vi "XW_Tutu_Chevray.vi"() -> (5 "Plug in titles":string[](array[string]), 7 "Plug in values":string[](array[string]))   [LabVIEW 2010]
uses:
  Globals/Meas_global.vi
  Controls/Analysis_type_Enum.ctl
  Controls/In_Range.ctl
  <vilib>/Utility/file.llb/Read From Spreadsheet File (string).vi
panel:
  out "Third":dbl format="%#.3f"
  out "Filename":string
  out "Third Component":path
  out "Info index":i32
  out "Log Row":i32
  out "2nd Comp":string
  out "1st Comp":string
  out "Iterations":i32
  out "Results table":string[][](table)
  out "Psi 2":dbl=-999.0 format="%.2f"
  out "Psi 1":dbl=-999.0 format="%.2f"
  out "UW":bool
  out "Indicies":i32[](array[numeric])
  in  "constants":T1={"u'/U"=0.5, "v'/U"=0.4, "w'/U"=0.4, "rho"=0.5, "alpha1"=0.0, "alpha2"=0.0} {"alpha2" format="%.2f"; "alpha1" format="%.2f"; "rho" format="%.2f"; "w'/U" format="%.2f"; "v'/U" format="%.2f"; "u'/U" format="%.2f"}
  in  "u*, v* limits":T2={"u* low"=0.4, "u* high"=1.8, "v* low"=-0.6, "v* high"=0.8} {"v* high" format="%.2f"; "v* low" format="%.2f"; "u* high" format="%.2f"; "u* low" format="%.2f"}
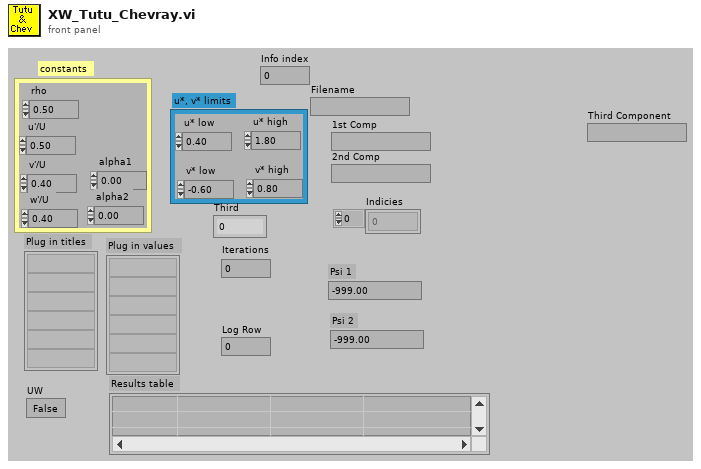
[diagram p1: front panel]
types:
  T1 = cluster{"u'/U":dbl, "v'/U":dbl, "w'/U":dbl, "rho":dbl, "alpha1":dbl, "alpha2":dbl}
  T2 = cluster{"u* low":dbl, "u* high":dbl, "v* low":dbl, "v* high":dbl}
  T3 = typedef "Correlation_cluster.ctl" = cluster{"U inst":string, "W inst":string, "uw":dbl, "uw/u'w'":dbl, "u^2w":dbl, "uw^2":dbl, "uw^3":dbl, "u^3w":dbl, "u^2w^2":dbl}
  T4 = typedef "Velocity_cluster.ctl" = cluster{"Name":string, "U":dbl, "u^2":dbl, "u^3/(u^2)^(1.5)":dbl, "u^4/(u^2)^2 -3":dbl, "% u'/U":dbl, "Mean % Err":dbl, "u^4":dbl}
  T5 = typedef "Analysis_type_cluster.ctl" = cluster{"Analysis type":T6, "Indicies":i32[], "Name":string, "Inst Array":T7, "Info index":i32}
  T6 = typedef "Analysis_type_Enum.ctl" = enum16{"Slow Response", "Fast Response", "Weighted Fast Response", "Fast FID", "Weighted Fast FID", "Cross Wire", "Weighted Cross Wire", "Weighted LDA"}
  T7 = typedef "Instrument_Array.ctl" = enum16{"PWA", "LDA", "Analogue"}
  T8 = typedef "In_Range.ctl" = enum16{"%", "±", "% & ±"}
  T9 = enum16{"Save no data", "Save data in new files", "Save data in existing files"}
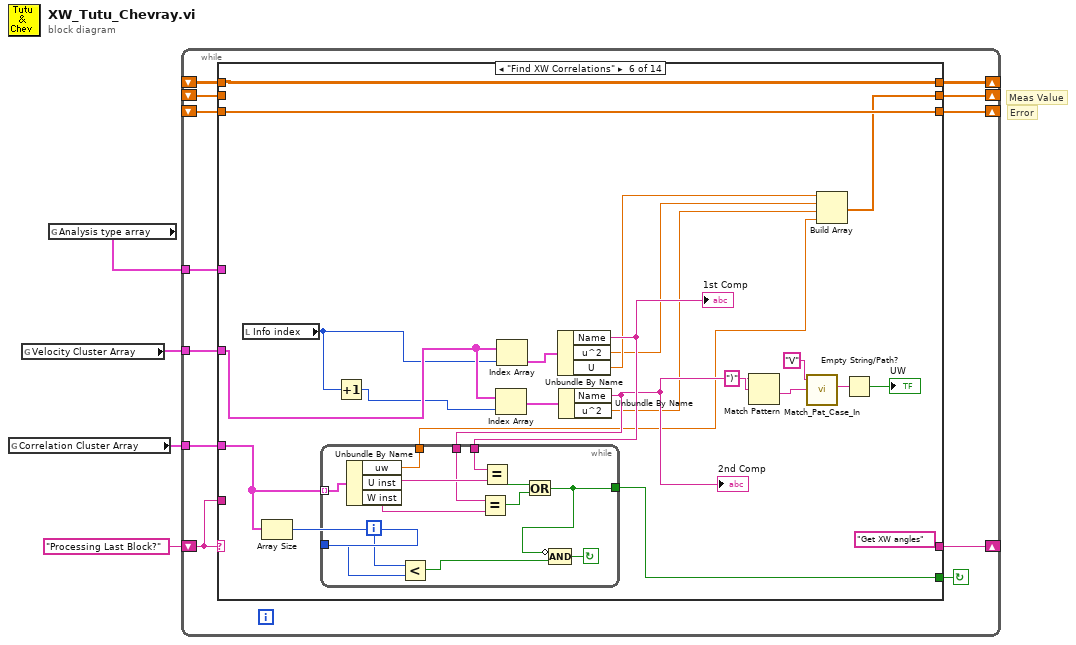
[diagram p0: block diagram]
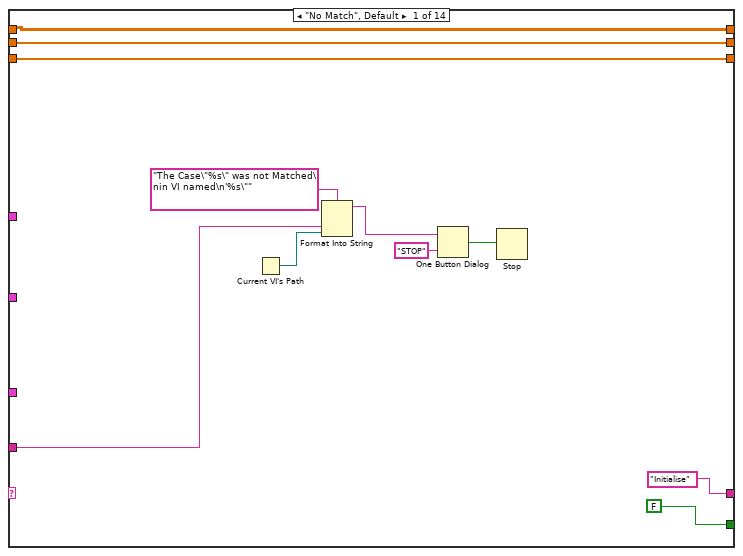
[diagram p2: hidden frame]
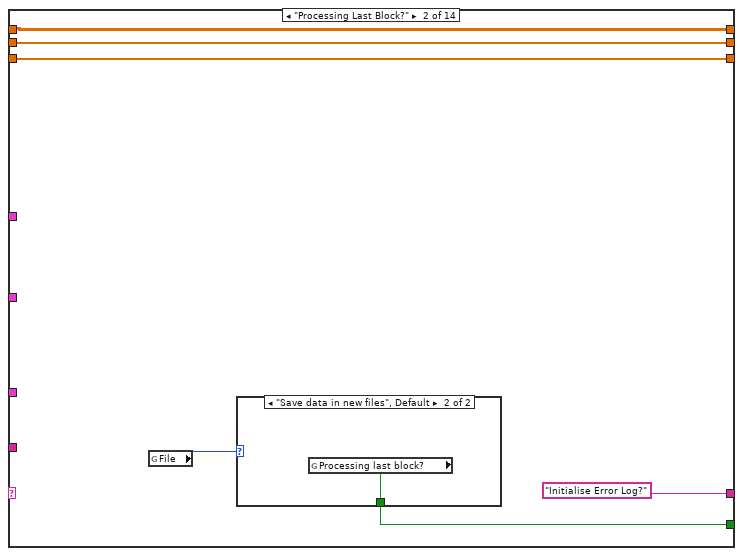
[diagram p3: hidden frame]
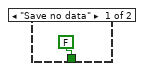
[diagram p4: hidden frame]
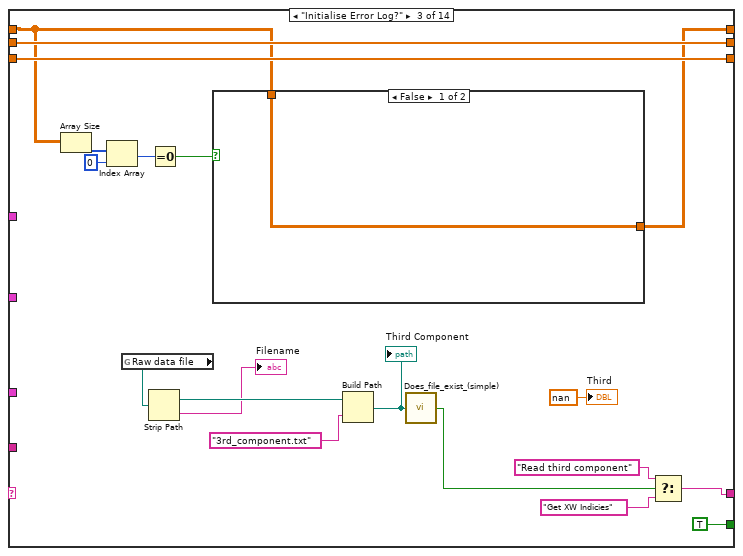
[diagram p5: hidden frame]
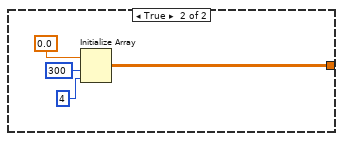
[diagram p6: hidden frame]
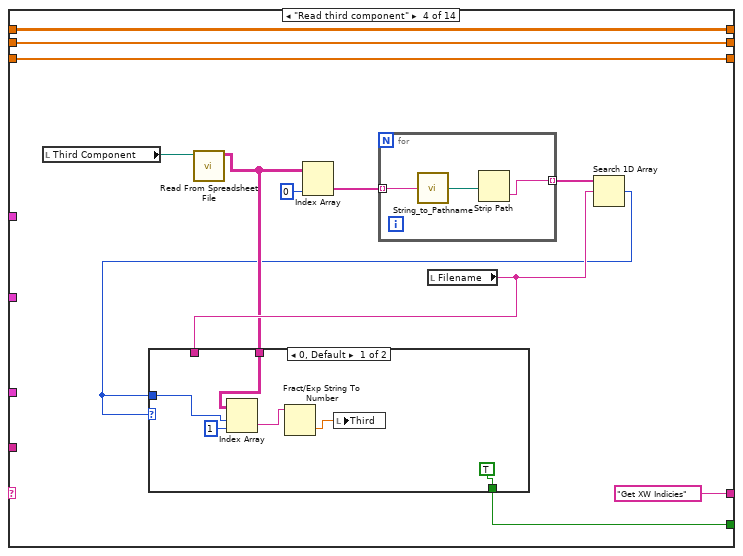
[diagram p7: hidden frame]
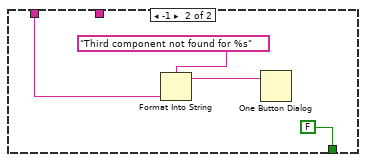
[diagram p8: hidden frame]
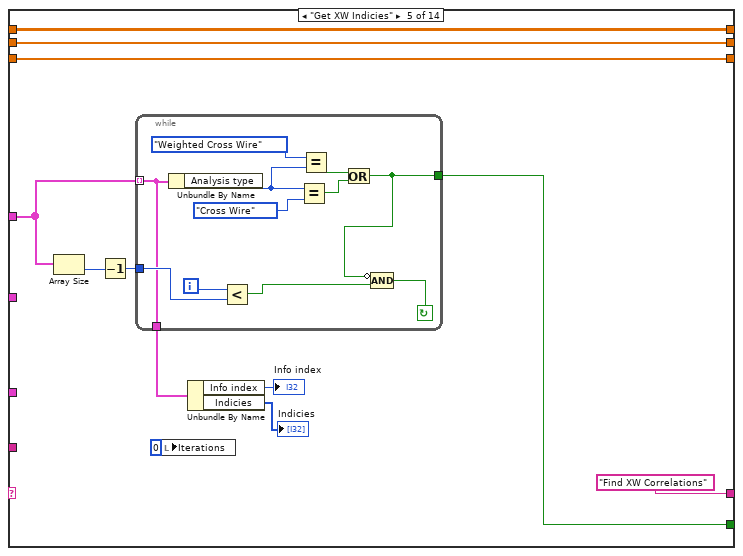
[diagram p9: hidden frame]
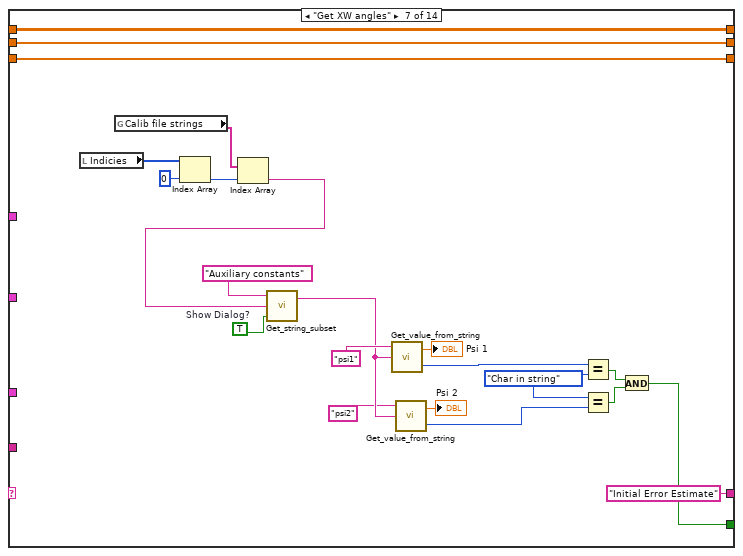
[diagram p10: hidden frame]
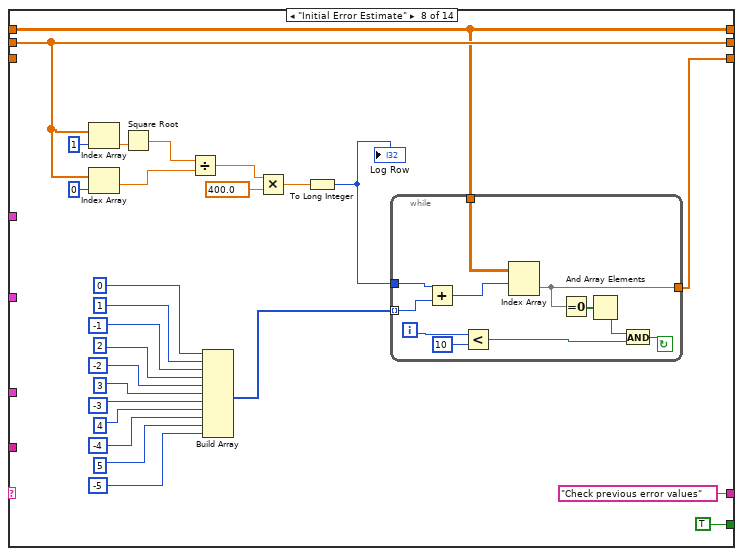
[diagram p11: hidden frame]
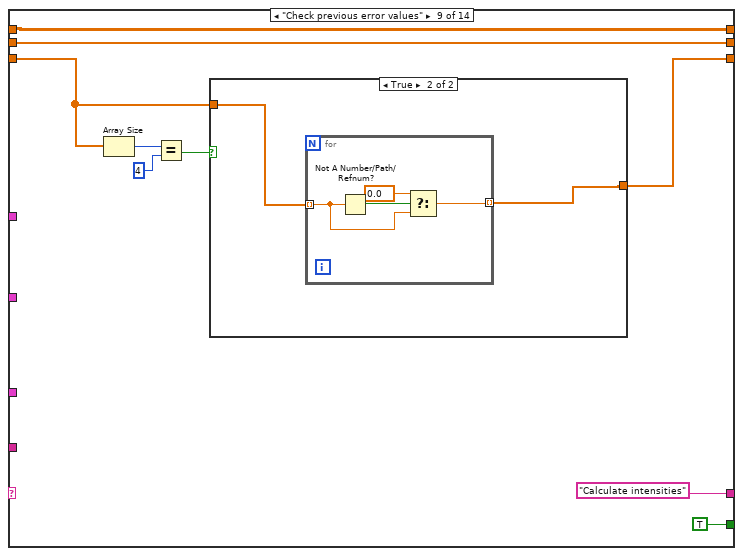
[diagram p12: hidden frame]
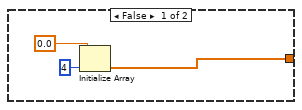
[diagram p13: hidden frame]
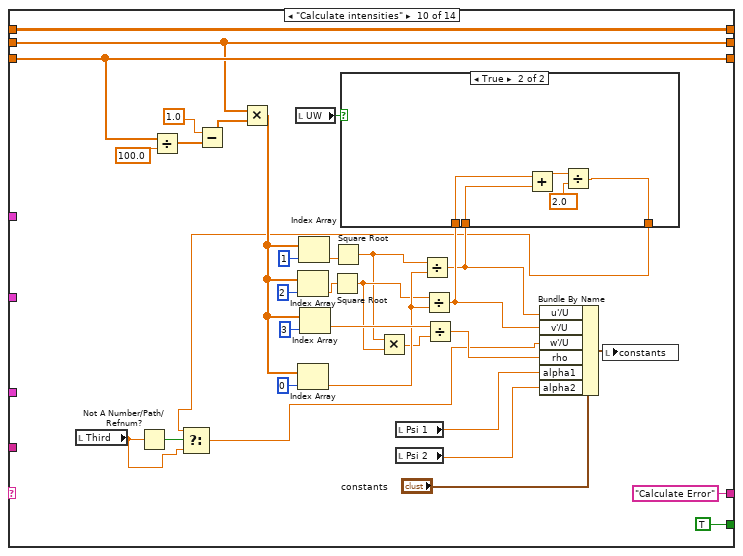
[diagram p14: hidden frame]
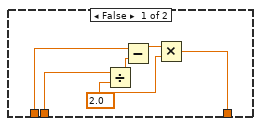
[diagram p15: hidden frame]
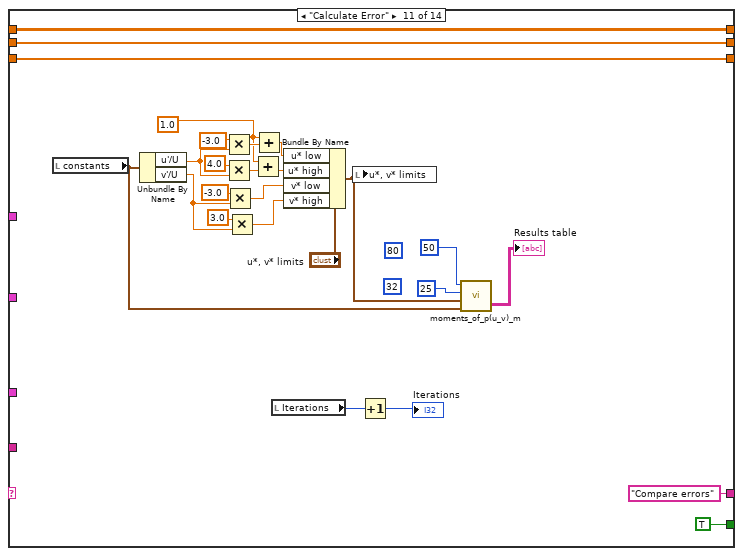
[diagram p16: hidden frame]
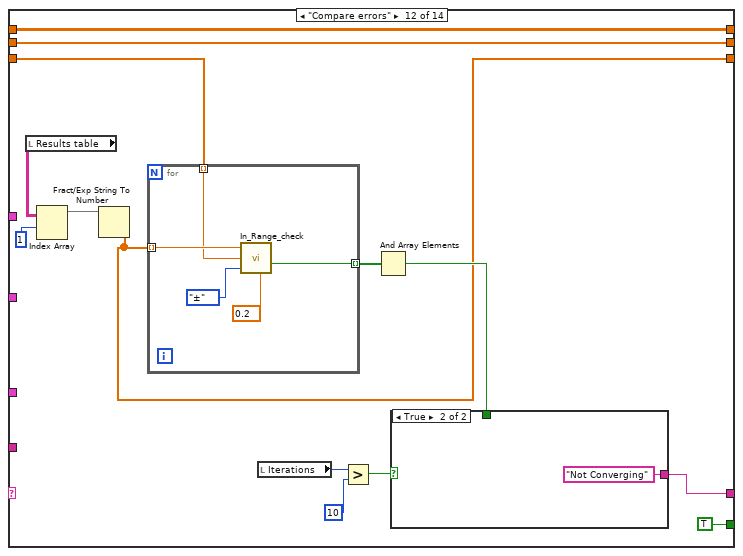
[diagram p17: hidden frame]
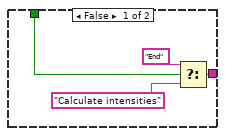
[diagram p18: hidden frame]
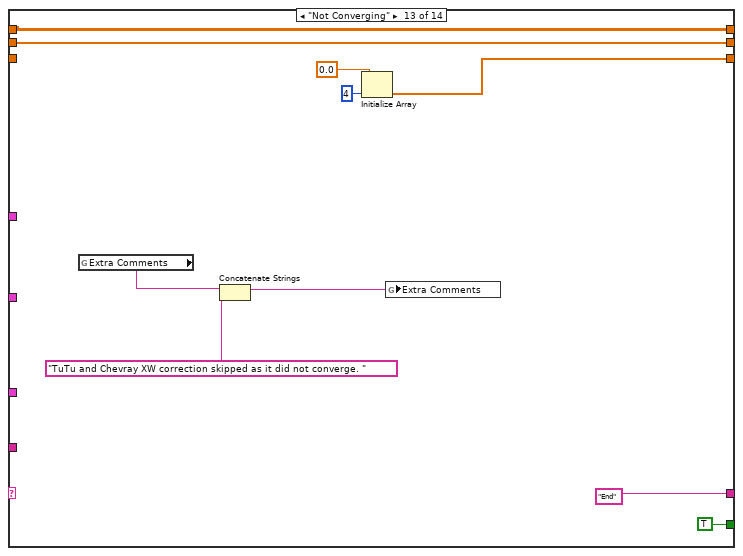
[diagram p19: hidden frame]
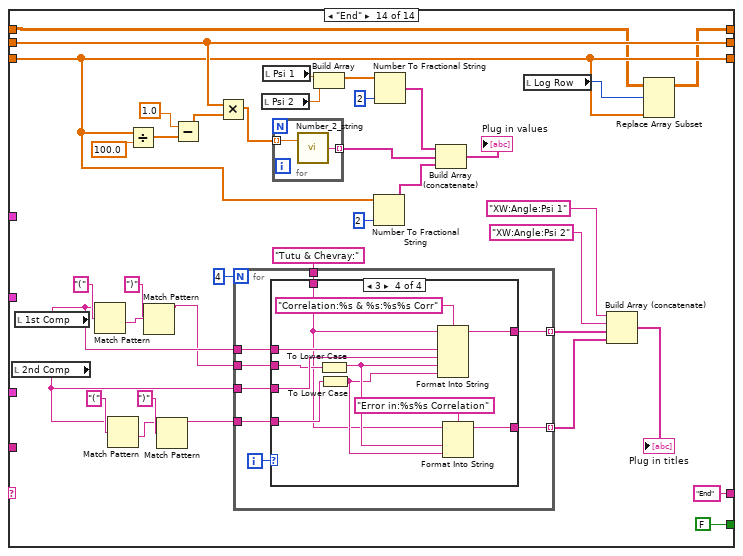
[diagram p20: hidden frame]
diagram:
  # "Error"
  # "Meas Value"
  n1 = global read "Meas_global.vi" "Correlation Cluster Array"() -> (w1:T3[])
  n2 = global read "Meas_global.vi" "Velocity Cluster Array"() -> (w2:T4[])
  n3 = global read "Meas_global.vi" "Analysis type array"() -> (w3:T5[])
  n4 = while {
    tunnel: w1 -> [w8]
    tunnel: w2 -> [w9]
    tunnel: w3 -> [w13]
    shift-left: _ -> [w7]
    shift-right: [w10] -> _
    shift-left: _ -> [w11]
    shift-right: [w12] -> _
    shift-left: "Processing Last Block?" -> [w14]
    shift-right: [w15] -> _
    shift-right: [w5] -> _
    shift-left: _ -> [w6]
    stop <- w16 continue-if-true
    n5 = case shown="\"Find XW Correlations\"" w14 {
      tunnel: [FALSE w32 TRUE ("Processing last block?") w62 w91 w111 w145 TRUE ("Processing last block?") TRUE ("Processing last block?") TRUE ("Processing last block?") TRUE ("Processing last block?") TRUE ("Processing last block?") TRUE ("Processing last block?") FALSE ("Processing last block?")] -> w16
      tunnel: ["Initialise" "Initialise Error Log?" w38 "Get XW Indicies" "Find XW Correlations" "Get XW angles" "Initial Error Estimate" "Check previous error values" ("f") "Calculate intensities" "Calculate Error" "Compare errors" w299 "End" "End"] -> w15
      tunnel: w14 -> [w22 _ _ _ _ _ _ _ _ _ _ _ _ _]
      tunnel: w13 -> [_ _ _ _ w95 _ _ _ _ _ _ _ _ _]
      tunnel: [w19 w31 w54 w70 w90 w116 w153 w184 w211 w245 w290 w304 w324 w356] -> w12
      tunnel: w11 -> [w19 w31 w54 w70 w90 _ w153 w184 w211 w245 w290 w304 w324 w356]
      tunnel: [w18 w29 w53 w69 w89 w129 w152 w178 w207 w250 w270 w295 w320 w329] -> w10
      tunnel: w9 -> [_ _ _ _ _ w126 _ _ _ _ _ _ _ _]
      tunnel: w8 -> [_ _ _ _ _ w125 _ _ _ _ _ _ _ _]
      tunnel: w7 -> [w18 w29 w53 w69 w89 w129 w152 _ w206 w250 w270 w302 _ w329]
      tunnel: [w17 w28 w47 w71 w88 w110 w144 w180 w204 w225 w265 w291 w315 w328] -> w5
      tunnel: w6 -> [w17 w28 w46 w71 w88 w110 w144 w180 w204 w225 w265 w291 w315 w327]
      frame "No Match", Default {
        n6 = Current VI's Path() -> (path=w21:path)
        n7 = Format Into String(format string="The Case\"%s\" was not Matched\nin VI named\n'%s\"" ("Format String"), w22, w21) -> (resulting string=w25:string)  [unwired: 2 in, 1 out]
        n8 = One Button Dialog(message=w25, button name ("OK")="STOP") -> (true=w23:bool)
        n9 = Stop(stop? (T)=w23) -> ()
      }
      frame "Processing Last Block?" {
        n10 = global read "Meas_global.vi" "File"() -> (w30:T9)
        n11 = case shown="\"Save data in new files\", Default" w30 {
          tunnel: [FALSE ("Processing last block?") w35] -> w32
          frame "Save no data" {
          }
          frame "Save data in new files", Default {
            n12 = global read "Meas_global.vi" "Processing last block?"() -> (w35:bool)
          }
        }
      }
      frame "Initialise Error Log?" {
        n13 = Array Size(array=w46) -> (size(s)=w51:i32[])
        n14 = Index Array(array=w51, index=0) -> (element=w49:i32)
        n15 = global read "Meas_global.vi" "Raw data file"() -> (w45:path)
        n16 = Strip Path(path=w45) -> (stripped path=w44:path, name=→"Filename":string)
        n17 = Equal To 0?(x=w49) -> (x = 0?=w48:bool)
        n18 = case shown="False" w48 {
          tunnel: [w55 w56] -> w47
          tunnel: w46 -> [w55 _]
          frame False {
          }
          frame True {
            n19 = Initialize Array(0.0, 300 ("dimension size"), 4 ("dimension size")) -> (w56:dbl[][])
          }
        }
        n20 = Build Path(base path=w44, name or relative path="3rd_component.txt") -> (appended path=w42:path)
        "Third Component" <- w42
        n21 = call "Does_file_exist_(simple).vi"("Pathname"=w42) -> ("exists?"=w39:bool)
        n22 = Select(t="Read third component", s=w39, f="Get XW Indicies") -> (s? t:f=w38:string)
        "Third" <- nan ("Third")
      }
      frame "Read third component" {
        n23 = local read "Third Component"() -> (w67:path)
        n24 = call-poly <vilib>:"Read From Spreadsheet File.vi"("file path (dialog if empty)"=w67) -> ("all rows"=w61:string[][])  [unwired: 3 in, 7 out]
        n25 = Index Array(array=w61, index (col)=0 ("disabled index (col)")) -> (element=w65:string[])  [unwired: 1 in]
        n26 = for {
          tunnel: w65 -> [w84] mode=indexing
          tunnel: [w82] -> w64 mode=indexing
          n27 = call "String_to_Pathname.vi"("Input String"=w84) -> ("path"=w83:path)
          n28 = Strip Path(path=w83) -> (name=w82:string)  [unwired: 1 out]
        }
        n29 = local read "Filename"() -> (w63:string)
        n30 = Search 1D Array(1D array=w64, element=w63) -> (index of element=w60:i32)  [unwired: 1 out]
        n31 = case shown="0, Default" w60 {
          tunnel: w63 -> [_ w81]
          tunnel: [TRUE ("Processing last block?") FALSE ("Processing last block?")] -> w62
          tunnel: w61 -> [w75 _]
          tunnel: w60 -> [w74 _]
          frame 0, Default {
            n32 = Index Array(array=w75, index (row)=w74, index (col)=1 ("disabled index (col)")) -> (element=w73:string)
            n33 = Fract/Exp String To Number(string=w73) -> (number=w72:dbl)  [unwired: 4 out]
            n34 = local write "Third"(w72) -> ()
          }
          frame -1 {
            n35 = Format Into String(format string="Third component not found for %s" ("message"), w81) -> (resulting string=w79:string)  [unwired: 2 in, 1 out]
            n36 = One Button Dialog(message=w79) -> ()  [unwired: 2 out]
          }
        }
      }
      frame "Get XW Indicies" {
        n37 = Array Size(array=w95) -> (size(s)=w94:i32)
        n38 = Decrement(x=w94) -> (x-1=w93:i32)
        n39 = while {
          tunnel: [w97] -> w91
          tunnel: [w98] -> w92
          tunnel: w93 -> [w101]
          tunnel: w95 -> [w98] mode=indexing
          i -> [w102]
          stop <- w99 continue-if-true
          n40 = Unbundle By Name(w98) -> ("Analysis type"=w106:T6)
          n41 = Less?(x=w102, y=w101) -> (x < y?=w100:bool)
          n42 = Equal?(x=w106, y=Analysis_type_Enum."Cross Wire" ("Analysis type")) -> (x = y?=w104:bool)
          n43 = Equal?(x=Analysis_type_Enum."Weighted Cross Wire" ("Analysis type"), y=w106) -> (x = y?=w103:bool)
          n44 = Or(x=w103, y=w104) -> (x .or. y?=w97:bool)
          n45 = Compound Arithmetic op=AND(invert w97, w100) -> (w99:bool)
        }
        n46 = local write "Iterations"(0 ("Iterations")) -> ()
        n47 = Unbundle By Name(w92) -> ("Info index"=→"Info index":i32, "Indicies"=→"Indicies":i32[])
      }
      frame "Find XW Correlations" {
        n48 = local read "Info index"() -> (w109:i32)
        n49 = Array Size(array=w125) -> (size(s)=w123:i32)
        n50 = Increment(x=w109) -> (x+1=w108:i32)
        n51 = Index Array(array=w126, index=w108) -> (element=w127:T4)
        n52 = Index Array(array=w126, index=w109) -> (element=w128:T4)
        n53 = Unbundle By Name(w128) -> ("Name"=w124:string, "u^2"=w113:dbl, "U"=w115:dbl)
        "1st Comp" <- w124
        n54 = Unbundle By Name(w127) -> ("Name"=w121:string, "u^2"=w114:dbl)
        "2nd Comp" <- w121
        n55 = while {
          tunnel: [w131] -> w112
          tunnel: w121 -> [w132]
          tunnel: w124 -> [w133]
          tunnel: w125 -> [w136] mode=indexing
          tunnel: [w137] -> w111
          tunnel: w123 -> [w140]
          i -> [w141]
          stop <- w138 continue-if-true
          n56 = Unbundle By Name(w136) -> ("uw"=w131:dbl, "U inst"=w135:string, "W inst"=w134:string)
          n57 = Less?(x=w141, y=w140) -> (x < y?=w139:bool)
          n58 = Equal?(x=w132, y=w134) -> (x = y?=w143:bool)
          n59 = Equal?(x=w133, y=w135) -> (x = y?=w142:bool)
          n60 = Or(x=w142, y=w143) -> (x .or. y?=w137:bool)
          n61 = Compound Arithmetic op=AND(invert w137, w139) -> (w138:bool)
        }
        n62 = Match Pattern(string=w121, regular expression=")") -> (after substring=w119:string)  [unwired: 4 out]
        n63 = call "Match_Pat_Case_In.vi"("String to match"="V" ("regular expression"), "String"=w119) -> ("Matched string"=w118:string)  [unwired: 1 in, 3 out]
        n64 = Build Array(w115, w113, w114, w112) -> (w116:dbl[])
        n65 = Empty String/Path?(string/path=w118) -> (empty?=→"UW":bool)
      }
      frame "Get XW angles" {
        w150 = enum16{"Char in string", "Char not in string"}."Char in string" ("Status")
        w160 = TRUE  # Show Dialog?
        n66 = local read "Indicies"() -> (w164:i32[])
        n67 = global read "Meas_global.vi" "Calib file strings"() -> (w163:string[])
        n68 = Index Array(array=w164, index=0 ("Index")) -> (element=w162:i32)
        n69 = Index Array(array=w163, index=w162) -> (element=w159:string)
        n70 = call "Get_string_subset.vi"("Show Dialog?"=w160, "String to split"=w159, "File Label"="Auxiliary constants") -> ("Output string"=w157:string)  [unwired: 1 out]
        n71 = call "Get_value_from_string.vi"("Input string"=w157, "Variable name"="psi1") -> ("Status"=w149:enum16{"Char in string", "Char not in string"}, "Value"=→"Psi 1":dbl)  [unwired: 1 in]
        n72 = call "Get_value_from_string.vi"("Input string"=w157, "Variable name"="psi2") -> ("Status"=w148:enum16{"Char in string", "Char not in string"}, "Value"=→"Psi 2":dbl)  [unwired: 1 in]
        n73 = Equal?(x=w149, y=w150) -> (x = y?=w146:bool)
        n74 = Equal?(x=w150, y=w148) -> (x = y?=w147:bool)
        n75 = And(x=w146, y=w147) -> (x .and. y?=w145:bool)
      }
      frame "Initial Error Estimate" {
        n76 = Index Array(array=w184, index=1 ("Index")) -> (element=w186:dbl)
        n77 = Index Array(array=w184, index=0 ("Index")) -> (element=w182:dbl)
        n78 = Square Root(x=w186) -> (sqrt(x)=w183:dbl)
        n79 = Divide(x=w183, y=w182) -> (x/y=w181:dbl)
        n80 = Build Array(0, 1, -1, 2, -2, 3, -3, 4, -4, 5, -5) -> (w166:i32[])
        n81 = Multiply(x=w181, y=400.0) -> (x*y=w189:dbl)
        n82 = To Long Integer(number=w189) -> (32bit integer=w179:i32)
        "Log Row" <- w179
        n83 = while {
          tunnel: w180 -> [w202]
          tunnel: w179 -> [w201]
          tunnel: [w198] -> w178
          tunnel: w166 -> [w200] mode=indexing
          i -> [w194]
          stop <- w195 continue-if-true
          n84 = Add(x=w201, y=w200) -> (x+y=w199:i32)
          n85 = Less?(x=w194, y=10) -> (x < y?=w192:bool)
          n86 = Index Array(array=w202, index (row)=w199) -> (element=w198:dbl[])  [unwired: 1 in]
          n87 = Equal To 0?(x=w198) -> (x = 0?=w197:bool[])
          n88 = And Array Elements(Boolean array=w197) -> (logical AND=w196:bool)
          n89 = And(x=w196, y=w192) -> (x .and. y?=w195:bool)
        }
      }
      frame "Check previous error values" {
        n90 = Array Size(array=w206) -> (size(s)=w210:i32)
        n91 = Equal?(x=w210, y=4) -> (x = y?=w208:bool)
        n92 = case shown="True" w208 {
          tunnel: [w212 w215] -> w207
          tunnel: w206 -> [_ w216]
          frame False {
            n93 = Initialize Array(0.0, 4 ("Dimension Size")) -> (w212:dbl[])
          }
          frame True {
            n94 = for {
              tunnel: w216 -> [w218] mode=indexing
              tunnel: [w217] -> w215 mode=indexing
              n95 = Not A Number/Path/Refnum?(number/path/refnum=w218) -> (NaN/Path/Refnum?=w220:bool)
              n96 = Select(t=0.0, s=w220, f=w218) -> (s? t:f=w217:dbl)
            }
          }
        }
      }
      frame "Calculate intensities" {
        n97 = local read "Third"() -> (w221:dbl)
        n98 = Not A Number/Path/Refnum?(number/path/refnum=w221) -> (NaN/Path/Refnum?=w224:bool)
        n99 = Divide(x=w250, y=100.0) -> (x/y=w248:dbl[])
        n100 = Subtract(x=1.0, y=w248) -> (x-y=w246:dbl[])
        n101 = Multiply(x=w245, y=w246) -> (x*y=w239:dbl[])
        n102 = local read "UW"() -> (w230:bool)
        n103 = Index Array(array=w239, index=2 ("Index")) -> (element=w237:dbl)
        n104 = Index Array(array=w239, index=0 ("Index")) -> (element=w234:dbl)
        n105 = Index Array(array=w239, index=1 ("Index")) -> (element=w238:dbl)
        n106 = Index Array(array=w239, index=3 ("Index")) -> (element=w235:dbl)
        n107 = Square Root(x=w237) -> (sqrt(x)=w233:dbl)
        n108 = Square Root(x=w238) -> (sqrt(x)=w232:dbl)
        n109 = Multiply(x=w232, y=w233) -> (x*y=w231:dbl)
        n110 = local read "Psi 1"() -> (w251:dbl)
        n111 = local read "Psi 2"() -> (w252:dbl)
        n112 = Divide(x=w232, y=w234) -> (x/y=w228:dbl)
        n113 = Divide(x=w233, y=w234) -> (x/y=w229:dbl)
        n114 = case shown="True" w230 {
          tunnel: w229 -> [w255 w261]
          tunnel: w228 -> [w254 w260]
          tunnel: [w256 w262] -> w223
          frame False {
            w257 = 2.0 ("y")
            n115 = Divide(x=w254, y=w257) -> (x/y=w259:dbl)
            n116 = Subtract(x=w255, y=w259) -> (x-y=w258:dbl)
            n117 = Multiply(x=w258, y=w257) -> (x*y=w256:dbl)
          }
          frame True {
            n118 = Add(x=w261, y=w260) -> (x+y=w264:dbl)
            n119 = Divide(x=w264, y=2.0) -> (x/y=w262:dbl)
          }
        }
        n120 = Select(t=w223, s=w224, f=w221) -> (s? t:f=w222:dbl)
        n121 = Divide(x=w235, y=w231) -> (x/y=w236:dbl)
        n122 = Bundle By Name(cluster="constants", "u'/U"=w228, "v'/U"=w229, "w'/U"=w222, "rho"=w236, "alpha1"=w251, "alpha2"=w252) -> (w244:T1)
        n123 = local write "constants"(w244) -> ()
      }
      frame "Calculate Error" {
        (unwired) i16 32 ("grid size for z*")
        (unwired) i16 80 ("grid size for u* and v*")
        w277 = 1.0
        n124 = local read "constants"() -> (w273:T1)
        n125 = Unbundle By Name(w273) -> ("u'/U"=w279:dbl, "v'/U"=w278:dbl)
        n126 = Multiply(x=-3.0, y=w279) -> (x*y=w285:dbl)
        n127 = Multiply(x=4.0, y=w279) -> (x*y=w284:dbl)
        n128 = Multiply(x=-3.0, y=w278) -> (x*y=w281:dbl)
        n129 = Multiply(x=3.0, y=w278) -> (x*y=w280:dbl)
        n130 = Add(x=w277, y=w284) -> (x+y=w282:dbl)
        n131 = Add(x=w277, y=w285) -> (x+y=w283:dbl)
        n132 = local read "Iterations"() -> (w267:i32)
        n133 = Bundle By Name(cluster="u*, v* limits", "u* low"=w283, "u* high"=w282, "v* low"=w281, "v* high"=w280) -> (w272:T2)
        n134 = local write "u*, v* limits"(w272) -> ()
        n135 = Increment(x=w267) -> (x+1=→"Iterations":i32)
        n136 = call "moments_of_p(u_v)_m.vi"("constants"=w273, "u*, v* limits"=w272, "grid size for z*"=i16 25, "grid size for u* and v*"=i16 50) -> ("Results table"=→"Results table":string[][])  [unwired: 7 out]
      }
      frame "Compare errors" {
        n137 = local read "Results table"() -> (w296:string[][])
        n138 = Index Array(array=w296, index (row)=1) -> (element=w297:string[])  [unwired: 1 in]
        n139 = Fract/Exp String To Number(string=w297) -> (number=w295:dbl[])  [unwired: 4 out]
        n140 = for {
          tunnel: w295 -> [w313] mode=indexing
          tunnel: w302 -> [w312] mode=indexing
          tunnel: [w310] -> w303 mode=indexing
          n141 = call "In_Range_check.vi"("±"=0.2, "Mode"=In_Range."±", "Value"=w312, "Setpoint"=w313) -> ("In Range"=w310:bool)  [unwired: 1 in, 2 out]
        }
        n142 = local read "Iterations"() -> (w294:i32)
        n143 = Greater?(x=w294, y=10) -> (0:w292:bool)
        n144 = And Array Elements(Boolean array=w303) -> (logical AND=w301:bool)
        n145 = case shown="True" w292 {
          tunnel: w301 -> [w308 _]
          tunnel: [w306 "Not Converging" ("f")] -> w299
          frame False {
            n146 = Select(t="End", s=w308, f="Calculate intensities") -> (s? t:f=w306:string)
          }
          frame True {
          }
        }
      }
      frame "Not Converging" {
        n147 = global read "Meas_global.vi" "Extra Comments"() -> (w318:string)
        n148 = Concatenate Strings(w318, "TuTu and Chevray XW correction skipped as it did not converge. " ("Format String")) -> (w316:string)
        n149 = Initialize Array(0.0, 4 ("Dimension Size")) -> (w320:dbl[])
        n150 = global write "Meas_global.vi" "Extra Comments"(w316) -> ()
      }
      frame "End" {
        n151 = local read "2nd Comp"() -> (w343:string)
        n152 = local read "1st Comp"() -> (w348:string)
        n153 = Match Pattern(string=w348, regular expression="(") -> (after substring=w353:string)  [unwired: 4 out]
        n154 = Match Pattern(string=w343, regular expression="(") -> (after substring=w349:string)  [unwired: 4 out]
        n155 = Divide(x=w329, y=100.0) -> (x/y=w359:dbl[])
        n156 = Match Pattern(string=w353, regular expression=")") -> (before substring=w347:string)  [unwired: 4 out]
        n157 = Match Pattern(string=w349, regular expression=")") -> (before substring=w342:string)  [unwired: 4 out]
        n158 = Subtract(x=1.0, y=w359) -> (x-y=w357:dbl[])
        n159 = Multiply(x=w356, y=w357) -> (x*y=w326:dbl[])
        n160 = for {
          N: 4 -> [_]
          tunnel: "Tutu & Chevray:" -> [w371]
          tunnel: w348 -> [w370]
          tunnel: w347 -> [w369]
          tunnel: [w368] -> w346 mode=indexing
          tunnel: [w367] -> w345 mode=indexing
          tunnel: w343 -> [w366]
          tunnel: w342 -> [w365]
          i -> [w372]
          n161 = case shown="3" w372 {
            tunnel: w371 -> [w373 w381 w389 w397]
            tunnel: w370 -> [w376 w386 _ w402]
            tunnel: w369 -> [w379 w383 _ w400]
            tunnel: [w375 w385 w394 w405] -> w368
            tunnel: [w374 w384 w393 w404] -> w367
            tunnel: w366 -> [_ _ w391 w401]
            tunnel: w365 -> [_ _ w390 w403]
            frame 0, Default {
              n162 = To Upper Case(1:w379) -> (0:w380:string)
              n163 = Format Into String(format string="Mean:%s:%s Corr" ("Format String"), initial string=w373, w376, w380) -> (resulting string=w374:string)  [unwired: 1 in, 1 out]
              n164 = Format Into String(format string="Error in:%s Mean" ("Format String"), initial string=w373, w376) -> (resulting string=w375:string)  [unwired: 1 in, 1 out]
            }
            frame 1 {
              n165 = To Lower Case(string=w383) -> (all lower case string=w382:string)
              n166 = Format Into String(format string="Variance:%s:%s^2 Corr" ("Format String"), initial string=w381, w386, w382) -> (resulting string=w384:string)  [unwired: 1 in, 1 out]
              n167 = Format Into String(format string="Error in:%s Variance" ("Format String"), initial string=w381, w386) -> (resulting string=w385:string)  [unwired: 1 in, 1 out]
            }
            frame 2 {
              n168 = To Lower Case(string=w390) -> (all lower case string=w392:string)
              n169 = Format Into String(format string="Variance:%s:%s^2 Corr" ("Format String"), initial string=w389, w391, w392) -> (resulting string=w393:string)  [unwired: 1 in, 1 out]
              n170 = Format Into String(format string="Error in:%s Variance" ("Format String"), initial string=w389, w391) -> (resulting string=w394:string)  [unwired: 1 in, 1 out]
            }
            frame 3 {
              n171 = To Lower Case(string=w400) -> (all lower case string=w399:string)
              n172 = To Lower Case(string=w403) -> (all lower case string=w398:string)
              n173 = Format Into String(format string="Correlation:%s & %s:%s%s Corr" ("Format String"), initial string=w397, w402, w401, w399, w398) -> (resulting string=w404:string)  [unwired: 1 in, 1 out]
              n174 = Format Into String(format string="Error in:%s%s Correlation" ("Format String"), initial string=w397, w399, w398) -> (resulting string=w405:string)  [unwired: 1 in, 1 out]
            }
          }
        }
        n175 = local read "Psi 2"() -> (w333:dbl)
        n176 = local read "Psi 1"() -> (w334:dbl)
        n177 = for {
          tunnel: w326 -> [w364] mode=indexing
          tunnel: [w363] -> w325 mode=indexing
          n178 = call "Number_2_string.vi"("number"=w364) -> ("String"=w363:string)  [unwired: 1 in]
        }
        n179 = Build Array(w334, w333) -> (w332:dbl[])
        n180 = Number To Fractional String(number=w329, precision (6)=i16 2) -> (F-format string=w339:string[])  [unwired: 2 out]
        n181 = Number To Fractional String(number=w332, precision (6)=i16 2) -> (F-format string=w331:string[])  [unwired: 2 out]
        n182 = Build Array (concatenate)(w331, w325, w339) -> (→"Plug in values":string[])
        n183 = local read "Log Row"() -> (w330:i32)
        n184 = Build Array (concatenate)("XW:Angle:Psi 1", "XW:Angle:Psi 2", w345, w346) -> (→"Plug in titles":string[])
        n185 = Replace Array Subset(array=w327, new element=w329, index (row)=w330) -> (w328:dbl[][])  [unwired: 1 in]
      }
    }
  }
